vi "Combine xml files.vi"() -> ()   [LabVIEW 2020]
uses:
  <vilib>/Utility/xml.llb/Read From XML File(array).vi
  <vilib>/Utility/xml.llb/Write to XML File(array).vi
panel:
  out "error out":errorcluster
  in  "path":path=path "C:/Users/niko.kuusniemi/temp/210419 HAST screen 3776 w2 no pull-up"
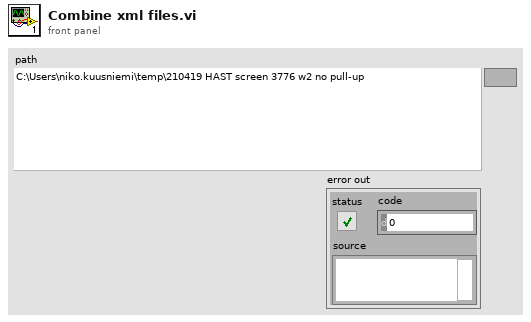
[diagram p1: front panel]
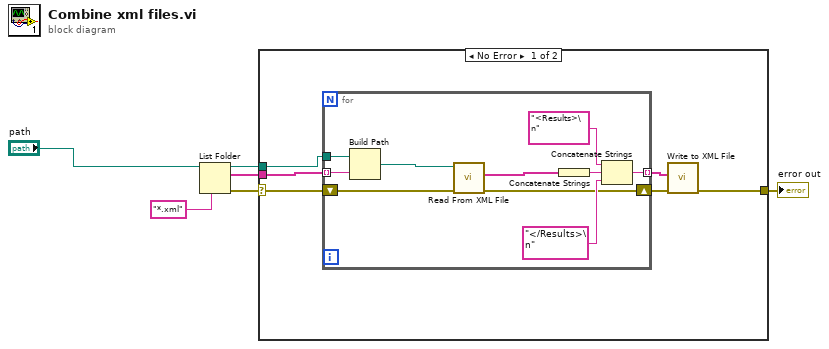
[diagram p0: block diagram]
diagram:
  n1 = List Folder(path="path", pattern="*.xml") -> (path out=w4:path, filenames=w3:string[], error out=w2:errorcluster)  [unwired: 2 in, 1 out]
  n2 = case shown="No Error" w2 {
    selector: w2 -> [w8 w23]
    tunnel: w4 -> [w12 _]
    tunnel: w3 -> [w11 _]
    tunnel: [w7 w23] -> w1
    frame No Error {
      n3 = for {
        tunnel: w12 -> [w22]
        tunnel: w11 -> [w21] mode=indexing
        tunnel: [w19] -> w10 mode=indexing
        shift-right: [w14] -> w9
        shift-left: w8 -> [w13]
        n4 = Build Path(base path=w22, name or relative path=w21) -> (appended path=w20:path)
        n5 = call-poly <vilib>:"Read From XML File.vi"("error in (no error)"=w13, "XML File Path"=w20) -> ("error out"=w14:errorcluster, "XML Elements"=w16:string[])  [unwired: 7 in, 1 out]
        n6 = Concatenate Strings(w16) -> (w15:string)
        n7 = Concatenate Strings("<Results>\n" ("new element/subarray"), w15, "</Results>\n" ("new element/subarray")) -> (w19:string)
      }
      n8 = call-poly <vilib>:"Write to XML File.vi"("error in (no error)"=w9, "XML Input"=w10) -> ("error out"=w7:errorcluster)  [unwired: 7 in, 2 out]
    }
    frame Error {
    }
  }
  "error out" <- w1
